vi "_New.vi"(8 "error in (no error)":errorcluster, 10 "Configuration":string="{ \"name\": \"DMM\", \"file\": \"JMETestSolutions.Instrument.DMM.lvlibp\", \"type\":\"JMETestSolutions.Instrument.DMM.lvlibp:JMETestSolutions.Instrument.DMM.lvclass\", \"Config\": {\"Channel\": \"1\",\"Mode\": \"Voltage\",\"Range\": 100}}") -> (0 "error out":errorcluster, 3 "Instrument":T1)   [LabVIEW 2020, in "JMETestSolutions.Instrument.lvlib" / "JMETestSolutions.Instrument.lvclass"]
doc: "The _New VI is used to instantiate an instance of the class"
uses:
  JMETestSolutions.Instrument.lvclass
  Common/Typdefs/Named Instrument.ctl
  JMETestSolutions.Instrument.lvlib
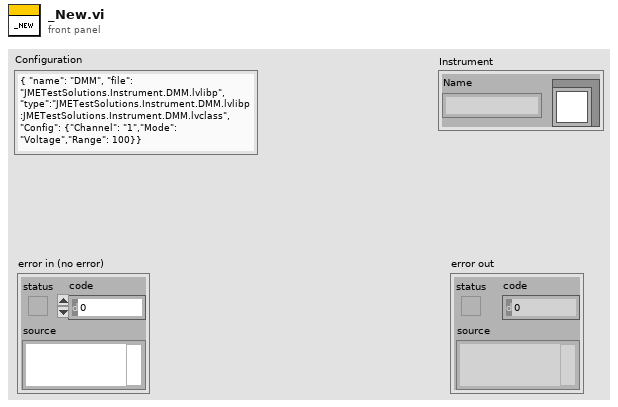
[diagram p1: front panel]
types:
  T1 = typedef "JMETestSolutions.Instrument.lvlib/Named Instrument.ctl" = cluster{"Name":string, "Instrument":refnum<class "JMETestSolutions.Instrument.lvclass">}
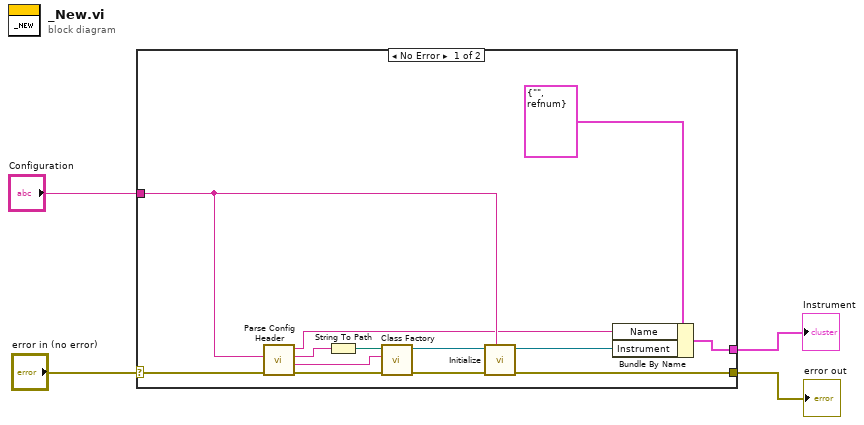
[diagram p0: block diagram]
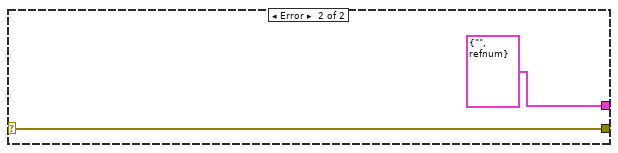
[diagram p2: hidden frame]
diagram:
  n1 = case shown="No Error" "error in (no error)" {
    selector: "error in (no error)" -> [w13 w19]
    tunnel: [w16 w19] -> w3
    tunnel: "Configuration" -> [w12 _]
    tunnel: [w14 T1 {"Name"="", "Instrument"=refnum} ("Instrument")] -> w1
    frame No Error {
      n2 = call "Parse Config Header.vi"("error in (no error)"=w13, "Config String"=w12) -> ("error out"=w11:errorcluster, "type"=w10:string, "file"=w5:string, "name"=w7:string)  [unwired: 6 in]
      n3 = String To Path(string=w5) -> (path=w6:path)
      n4 = call "Class Factory.vi"("error in (no error)"=w11, "ClassName"=w10, "FilePath"=w6) -> ("error out"=w17:errorcluster, "Instrument"=w9:refnum<class "JMETestSolutions.Instrument.lvclass">)  [unwired: 7 in]
      n5 = call-dynamic "Initialize.vi"("Configuration"=w12, "error in (no error)"=w17, "JMETestSolutions.Instrument in"=w9) -> ("error out"=w16:errorcluster, "JMETestSolutions.Instrument out"=w15:refnum<class "JMETestSolutions.Instrument.lvclass">)  [unwired: 7 in]
      n6 = Bundle By Name(cluster=T1 {"Name"="", "Instrument"=refnum} ("Instrument"), "Name"=w7, "Instrument"=w15) -> (w14:T1)
    }
    frame Error {
    }
  }
  "error out" <- w3
  "Instrument" <- w1
